vi "alarm map database.vi"(8 "error in (no error)":errorcluster, 11 "map in":T2) -> (0 "error out":errorcluster, 2 "change?":bool, 3 "map out":T1)   [LabVIEW 2022 SP3, in "Alarm interface.lvlib"]
uses:
  Alarm interface.lvlib
  <vilib>/addons/database/_DB Variant To Data/Database Variant To Data.xnode
panel:
  out "结果字符串":string
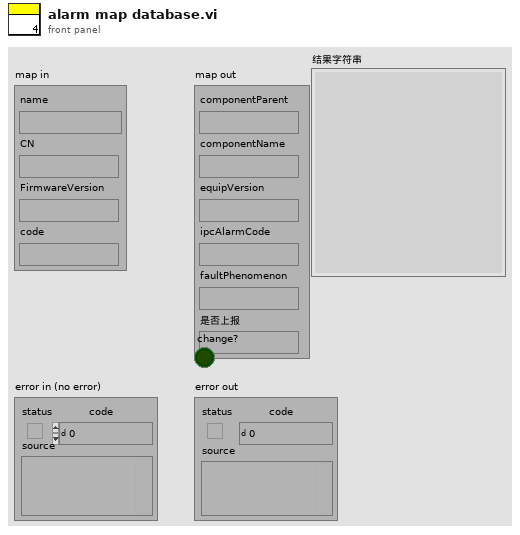
[diagram p1: front panel]
types:
  T1 = typedef "Alarm interface.lvlib/map out.ctl" = cluster{"componentParent":string, "componentName":string, "equipVersion":string, "ipcAlarmCode":string, "faultPhenomenon":string, "是否上报":string}
  T2 = typedef "Alarm interface.lvlib/map in.ctl" = cluster{"name":string, "CN":string, "FirmwareVersion":string, "code":string}
  T3 = cluster{"name":bool, "CN":bool, "FirmwareVersion":bool, "code":bool}
  T4 = cluster{"data[0]":string, "data[1]":string, "data[2]":string, "data[3]":string, "data[4]":string, "data[5]":string}
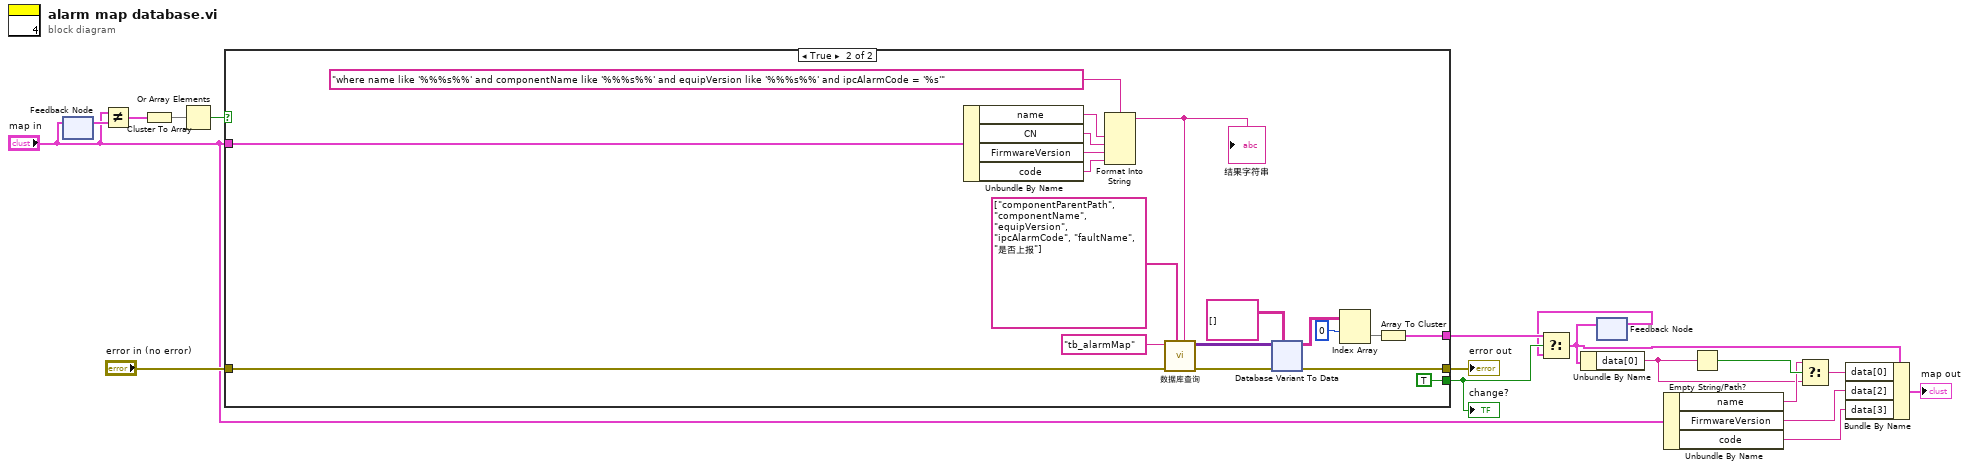
[diagram p0: block diagram]
diagram:
  n1 = feedback #1() -> (w18:T2)  [unwired: 1 in]
  n2 = feedback-in #1("map in") -> ()
  n3 = Not Equal?(x="map in", y=w18) -> (x != y?=w17:T3)
  n4 = Cluster To Array(cluster=w17) -> (array=w16:bool[])
  n5 = Or Array Elements(Boolean array=w16) -> (logical OR=w15:bool)
  n6 = case shown="True" w15 {
    tunnel: [_ w25] -> w14
    tunnel: "map in" -> [_ w23]
    tunnel: [_ TRUE] -> w13
    tunnel: "error in (no error)" -> [w19 w21]
    tunnel: [w19 w20] -> w10
    frame False {
    }
    frame True {
      n7 = Unbundle By Name(w23) -> ("name"=w33:string, "CN"=w31:string, "FirmwareVersion"=w30:string, "code"=w29:string)
      n8 = Format Into String(format string="where name like '%%%s%%' and componentName like '%%%s%%' and equipVersion like '%%%s%%' and ipcAlarmCode = '%s'" ("格式字符串"), w33, w31, w30, w29) -> (resulting string=w32:string)  [unwired: 2 in, 1 out]
      "结果字符串" <- w32
      n9 = call "数据库查询.vi"("condition"=w32, "columns"=string[] ["componentParentPath", "componentName", "equipVersion", "ipcAlarmCode", "faultName", "是否上报"], "error in (no error)"=w21, "table"="tb_alarmMap") -> ("error out"=w24:errorcluster, "data"=w36:variant[][])  [unwired: 5 in, 1 out]
      n10 = xnode "Database Variant To Data"("database variant"=w36, "error in (no error)"=w24, "type"=string[][] []) -> ("data"=w28:string[][], "error out"=w20:errorcluster)
      n11 = Index Array(array=w28, index (row)=0 ("索引 (行)")) -> (element=w26:string[])  [unwired: 1 in]
      n12 = Array To Cluster(array=w26) -> (cluster=w25:T4)
    }
  }
  "change?" <- w13
  "error out" <- w10
  n13 = feedback #2() -> (w12:T4)  [unwired: 1 in]
  n14 = Select(t=w14, s=w13, f=w12) -> (s? t:f=w5:T4)
  n15 = Unbundle By Name(w5) -> ("data[0]"=w2:string)
  n16 = feedback-in #2(w5) -> ()
  n17 = Unbundle By Name("map in") -> ("name"=w3:string, "FirmwareVersion"=w7:string, "code"=w6:string)
  n18 = Empty String/Path?(string/path=w2) -> (empty?=w4:bool)
  n19 = Select(t=w3, s=w4, f=w2) -> (s? t:f=w1:string)
  n20 = Bundle By Name(cluster=w5, "data[0]"=w1, "data[2]"=w7, "data[3]"=w6) -> (→"map out":T4)
